vi "ArrayToVector.vi"(11 "2D WF in":dbl[][](array[numeric])) -> (2 "WF Dimension":cluster{"NumOfWFs":i32, "WFLength":i32}, 3 "1D WF out":dbl[](array[numeric]))   [LabVIEW 2024]
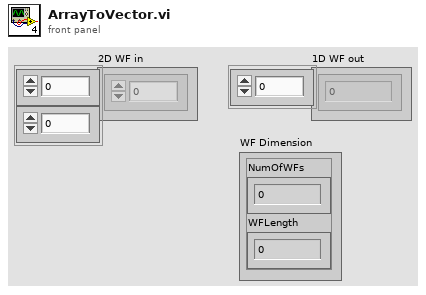
[diagram p1: front panel]
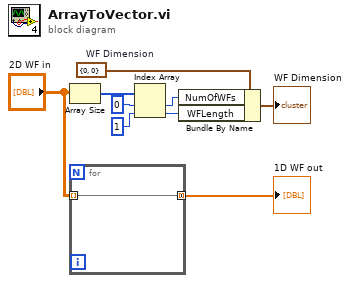
[diagram p0: block diagram]
diagram:
  w6 = cluster{"NumOfWFs":i32, "WFLength":i32} {"NumOfWFs"=0, "WFLength"=0}  # WF Dimension
  n1 = Array Size(array="2D WF in") -> (size(s)=w7:i32[])
  n2 = for {
    tunnel: "2D WF in" -> [w10] mode=indexing
    tunnel: [w10] -> w8 mode=concatenating
  }
  "1D WF out" <- w8
  n3 = Index Array(array=w7, index #1=0 ("index"), index #2=1 ("index")) -> (element #1=w3:i32, element #2=w2:i32)
  n4 = Bundle By Name(cluster=w6, "NumOfWFs"=w3, "WFLength"=w2) -> (→"WF Dimension":cluster{"NumOfWFs":i32, "WFLength":i32})
